vi "Write VI Name.vi"(8 "error in (no error)":errorcluster, 10 "VI Name":string, 11 "Tagbus PID Module configuration in":refnum<class "Tagbus PID Module configuration.lvclass">) -> (0 "error out":errorcluster, 3 "Tagbus PID Module configuration out":refnum<class "Tagbus PID Module configuration.lvclass">)   [LabVIEW 2014]
uses:
  Tagbus PID Module configuration.lvclass
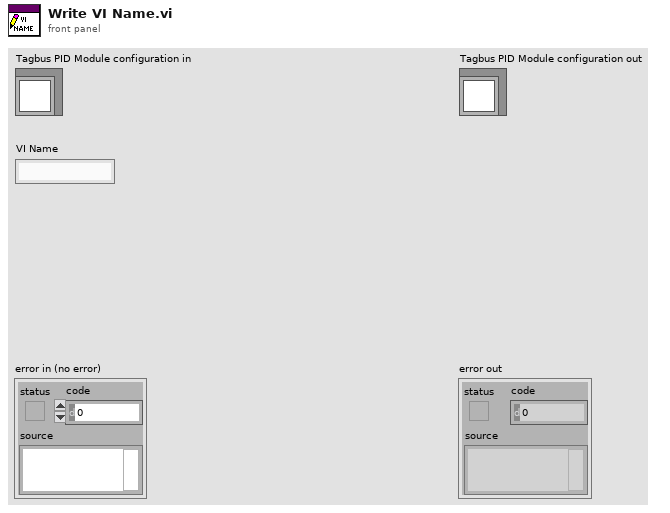
[diagram p1: front panel]
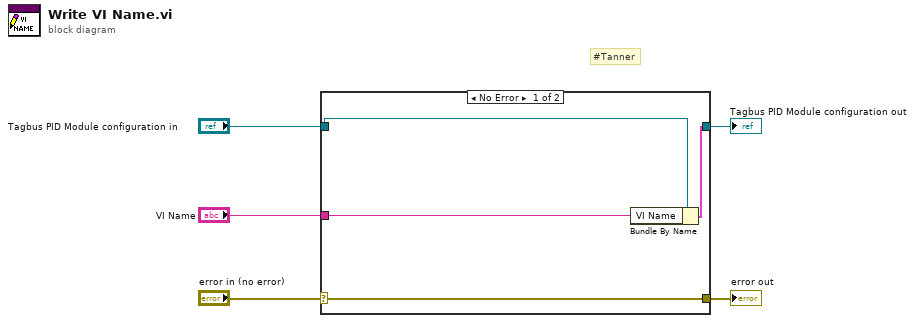
[diagram p0: block diagram]
diagram:
  # "#Tanner"
  n1 = case shown="No Error" "error in (no error)" {
    selector: "error in (no error)" -> [w9 w10]
    tunnel: [w9 w10] -> w4
    tunnel: [w7 w11] -> w2
    tunnel: "Tagbus PID Module configuration in" -> [w8 w11]
    tunnel: "VI Name" -> [w6 _]
    frame No Error {
      n2 = Bundle By Name(cluster=w8, "VI Name"=w6) -> (w7:cluster{})
    }
    frame Error {
    }
  }
  "error out" <- w4
  "Tagbus PID Module configuration out" <- w2
